vi "Report.vi"() -> ()   [LabVIEW 2017]
uses:
  <vilib>/Utility/miscctls.llb/LVRowAndColumnTypeDef.ctl
  <vilib>/Utility/miscctls.llb/LVRowAndColumnUnsignedTypeDef.ctl
  a160b8e7-0040-4e34-a052-5f80b3aab475.vi
  <vilib>/addons/database/Connection.llb/DB Tools Open Connec (String).vi
  <vilib>/Utility/file.llb/Write Delimited Spreadsheet (string).vi
  Global/Global 1.vi
  <vilib>/regexp/Match Regular Expression.xnode
  <vilib>/addons/database/NI_Database_API.lvlib
  <vilib>/Utility/NIReport.llb/NI_report.lvclass
  <vilib>/Utility/NIReport.llb/Append Text Table to Report (wrap).vi
panel:
  out "reposr save header":string[](array[string])
  in  "SELECT REPORT TYPE":string(combo)="WITH TRECIABILITY"
  out "error out":errorcluster
  in  "error in (no error)":errorcluster
  in  "GET REPORT":bool
  in  "EXIT":bool
  in  "EXPORT TO EXCEL":bool
  in  "TO":timestamp format="%<%x>T"
  in  "FROM":timestamp format="%<%x>T"
  in  "BARCODE":string
  in  "TYPE":string(combo)="DATE TIME"
  in  "STATION WISE":string(combo)="0"
  out "Table":string[][](table)
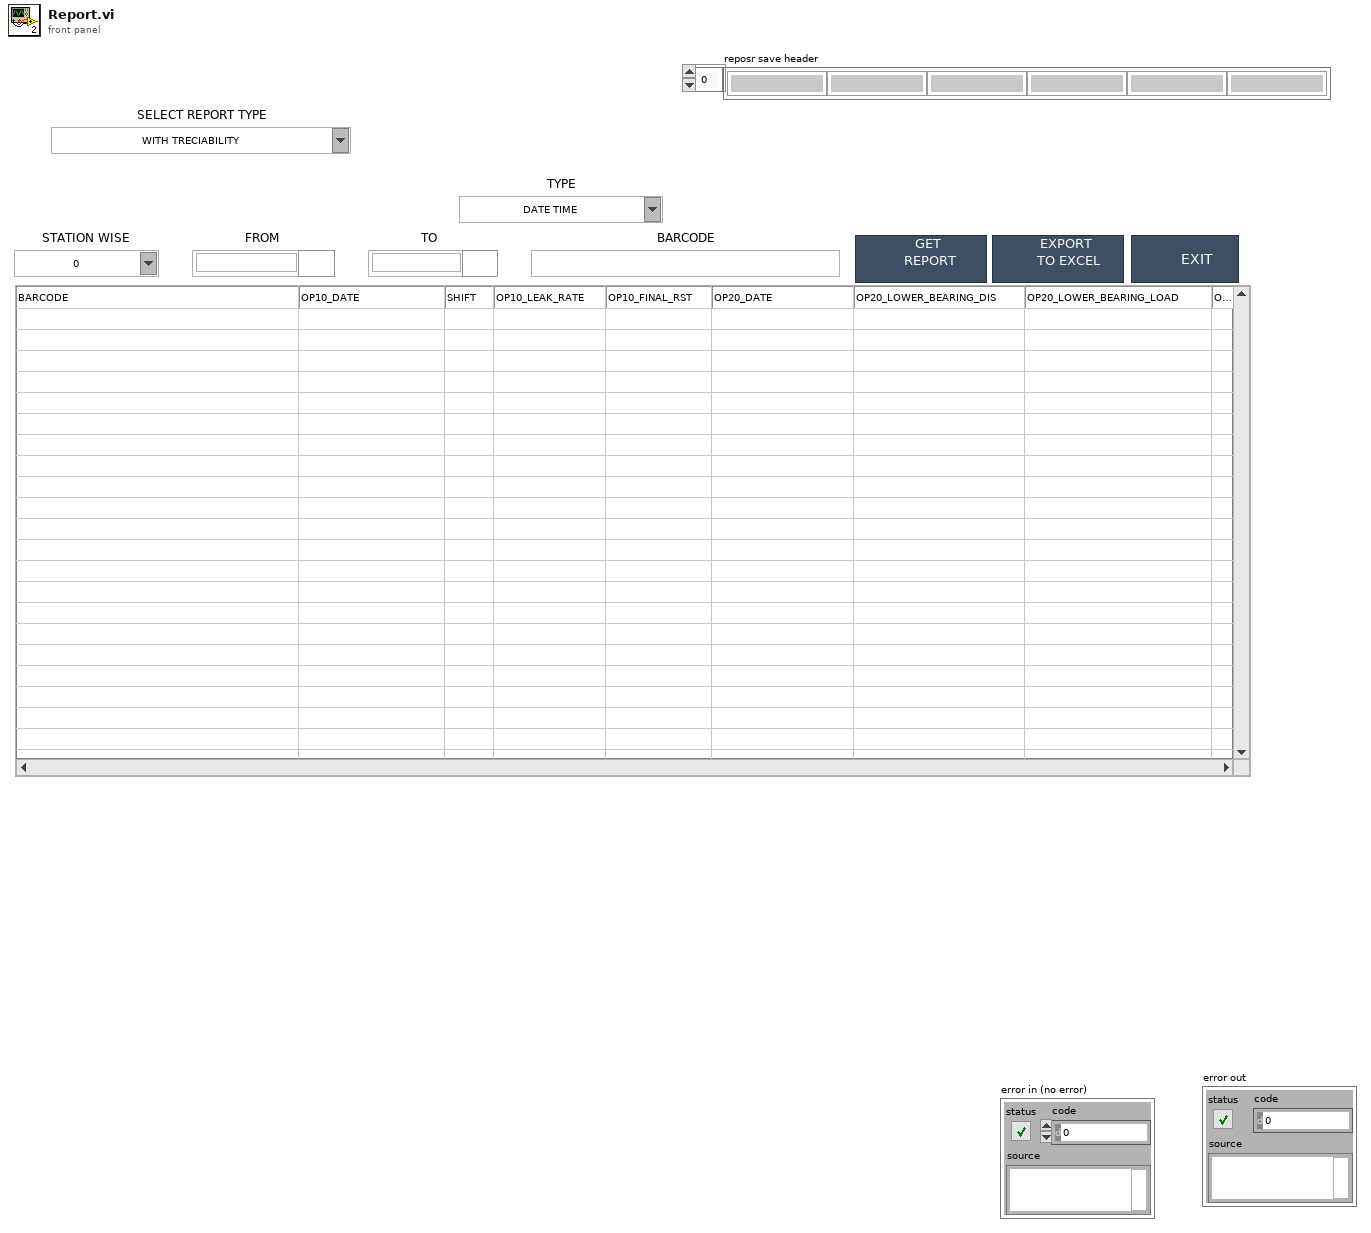
[diagram p1: front panel]
types:
  T1 = typedef "NI_Database_API.lvlib/Conn ObjectReference.ctl" = refnum<k1>
  T2 = typedef "LVRowAndColumnTypeDef.ctl" = cluster{"Row":i32, "Column":i32}
  T3 = typedef "LVRowAndColumnUnsignedTypeDef.ctl" = cluster{"Row":u32, "Column":u32}
  T4 = enum16{"Standard Report", "HTML", "Word", "Excel"}
  T5 = enum16{"maximized", "minimized", "normal", "no change"}
  T6 = enum32{"invalid app kind", "Development System", "Run Time System", "Student Edition", "Embedded LabVIEW", "Evaluation", "Custom"}
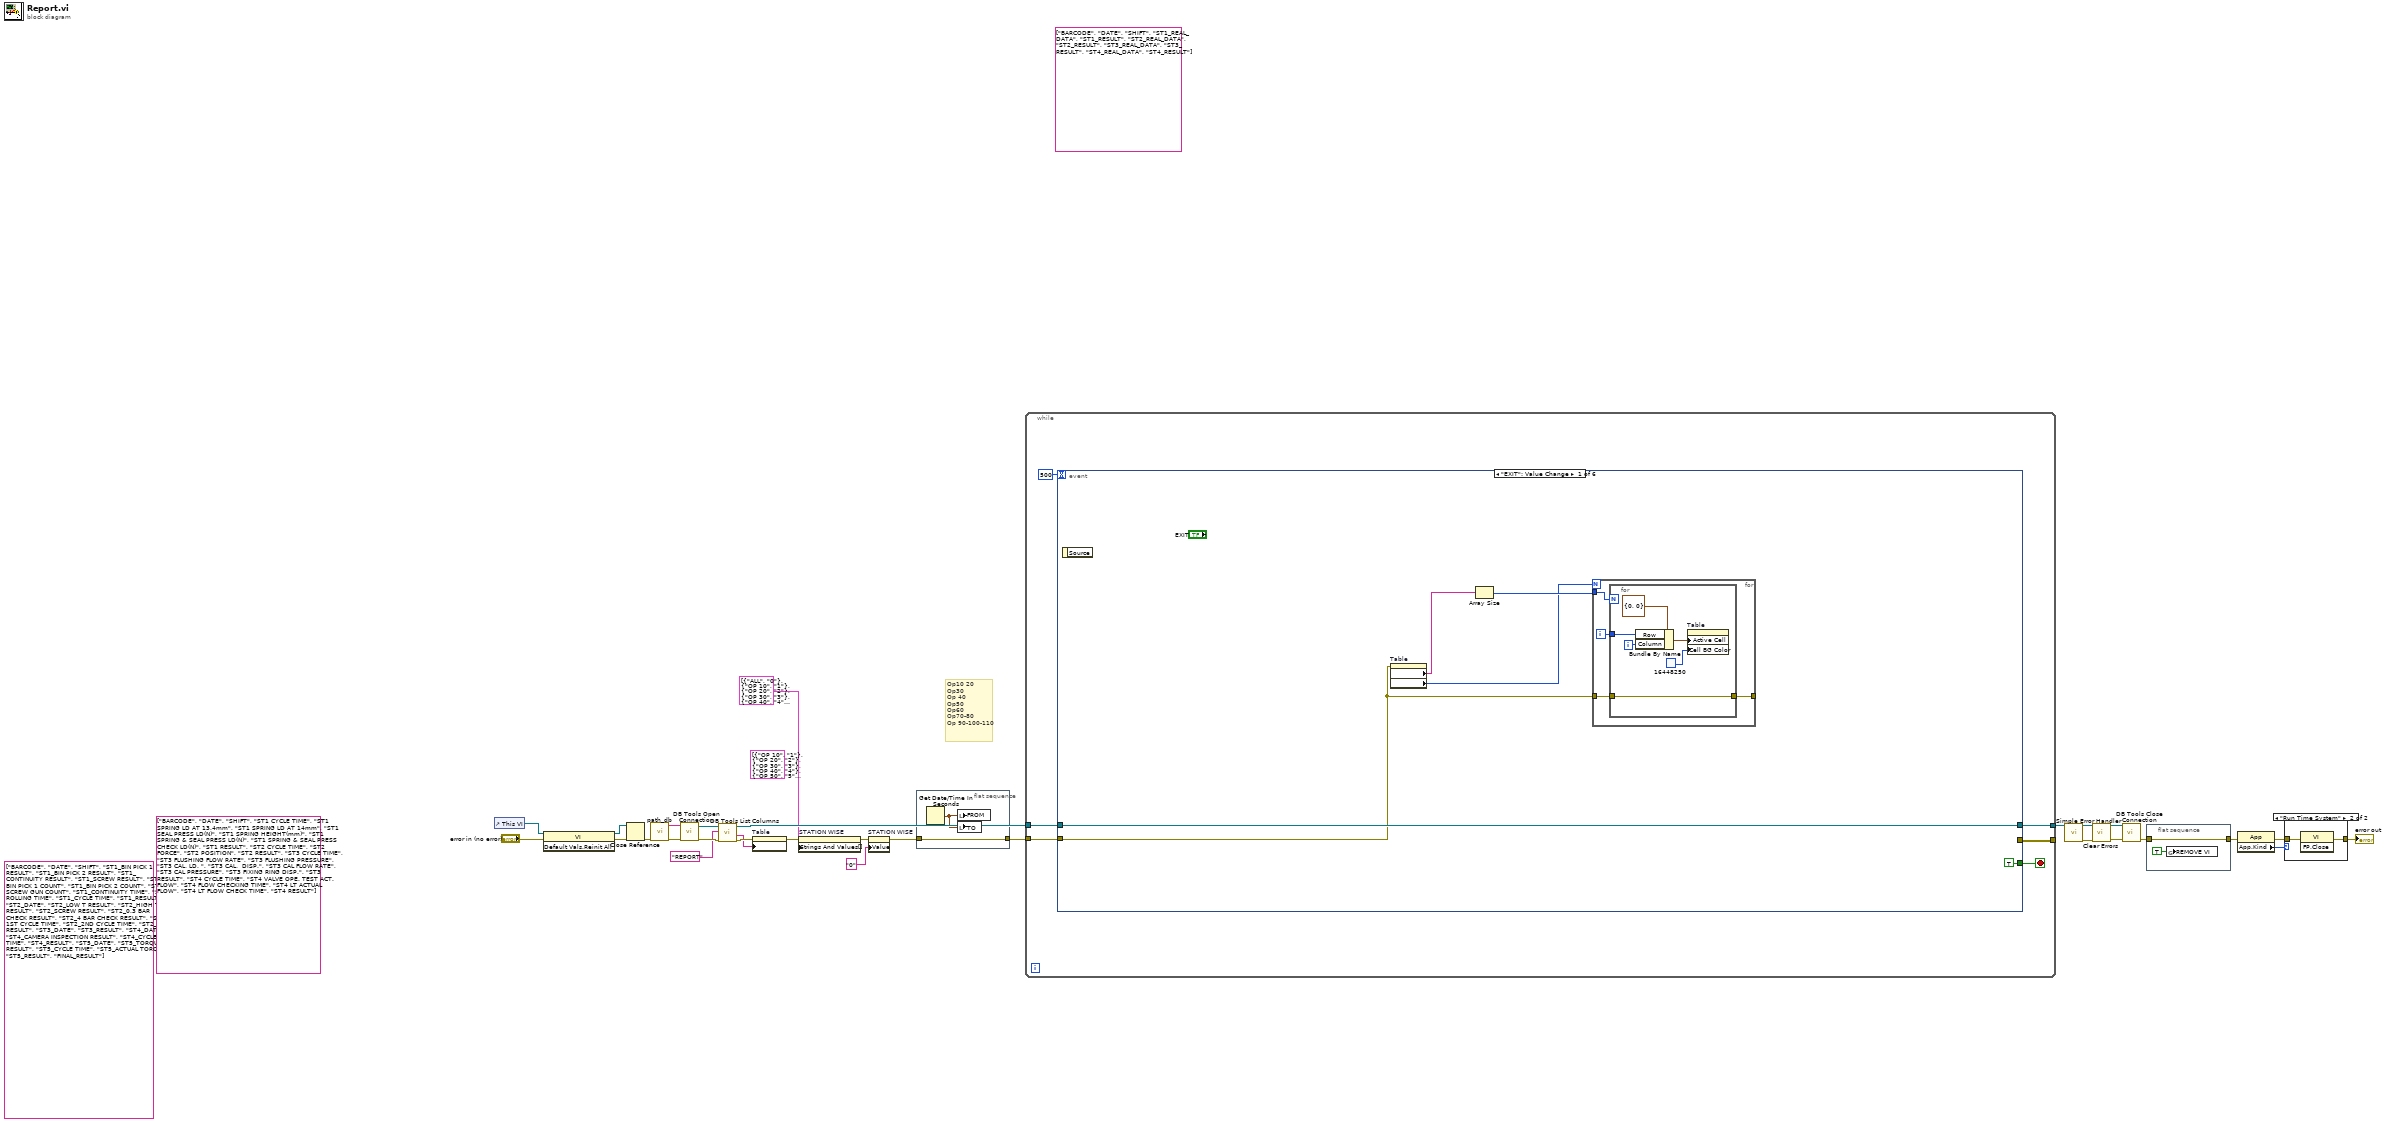
[diagram p0: block diagram]
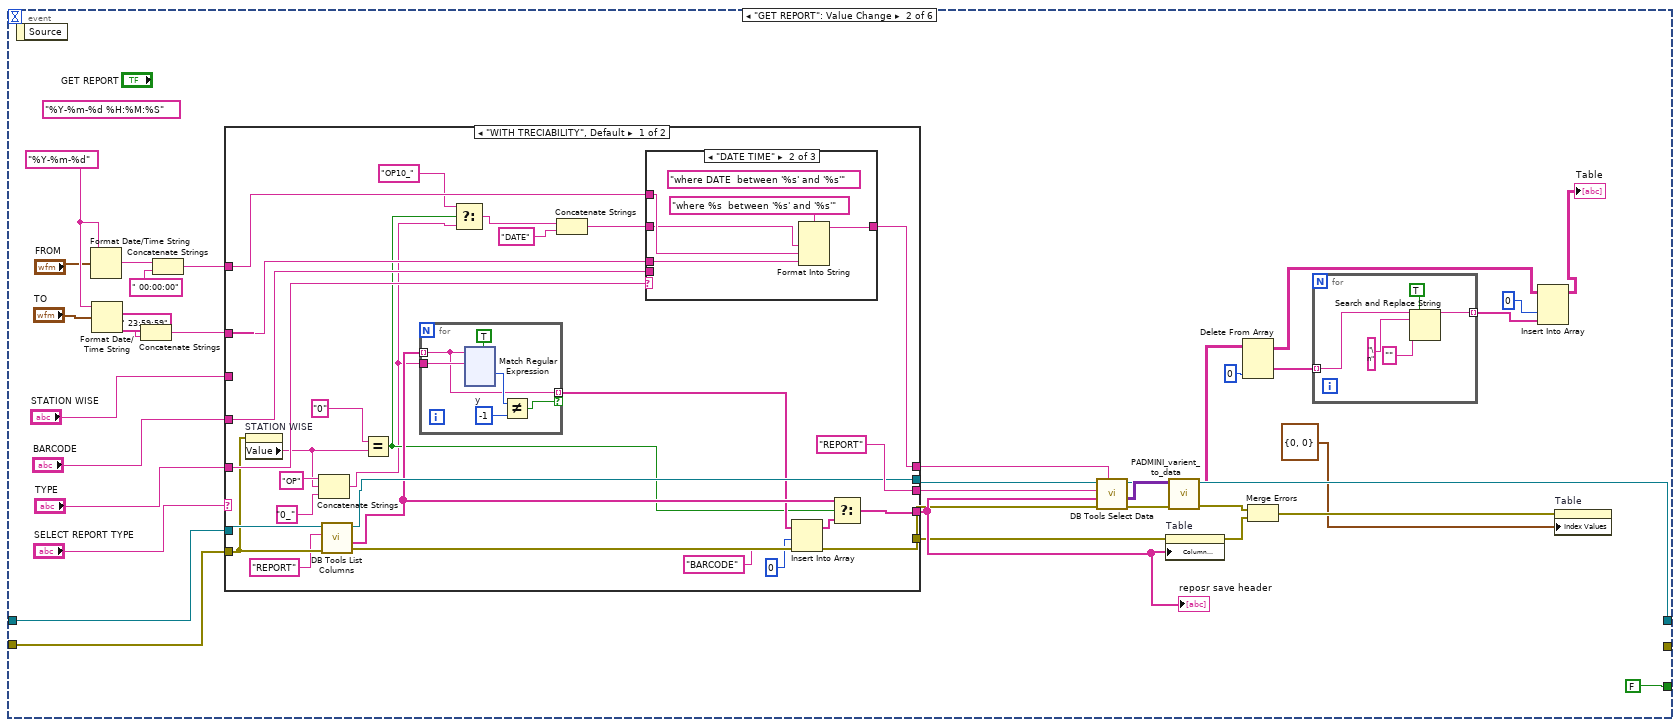
[diagram p2: hidden frame]
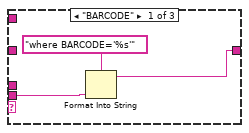
[diagram p3: hidden frame]
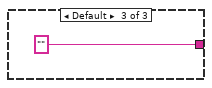
[diagram p4: hidden frame]
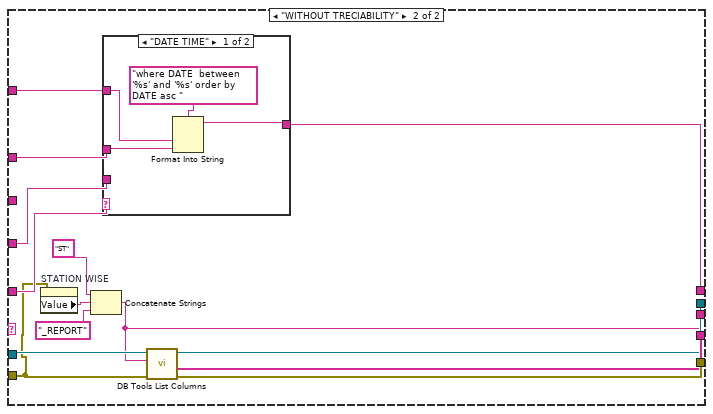
[diagram p5: hidden frame]
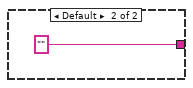
[diagram p6: hidden frame]
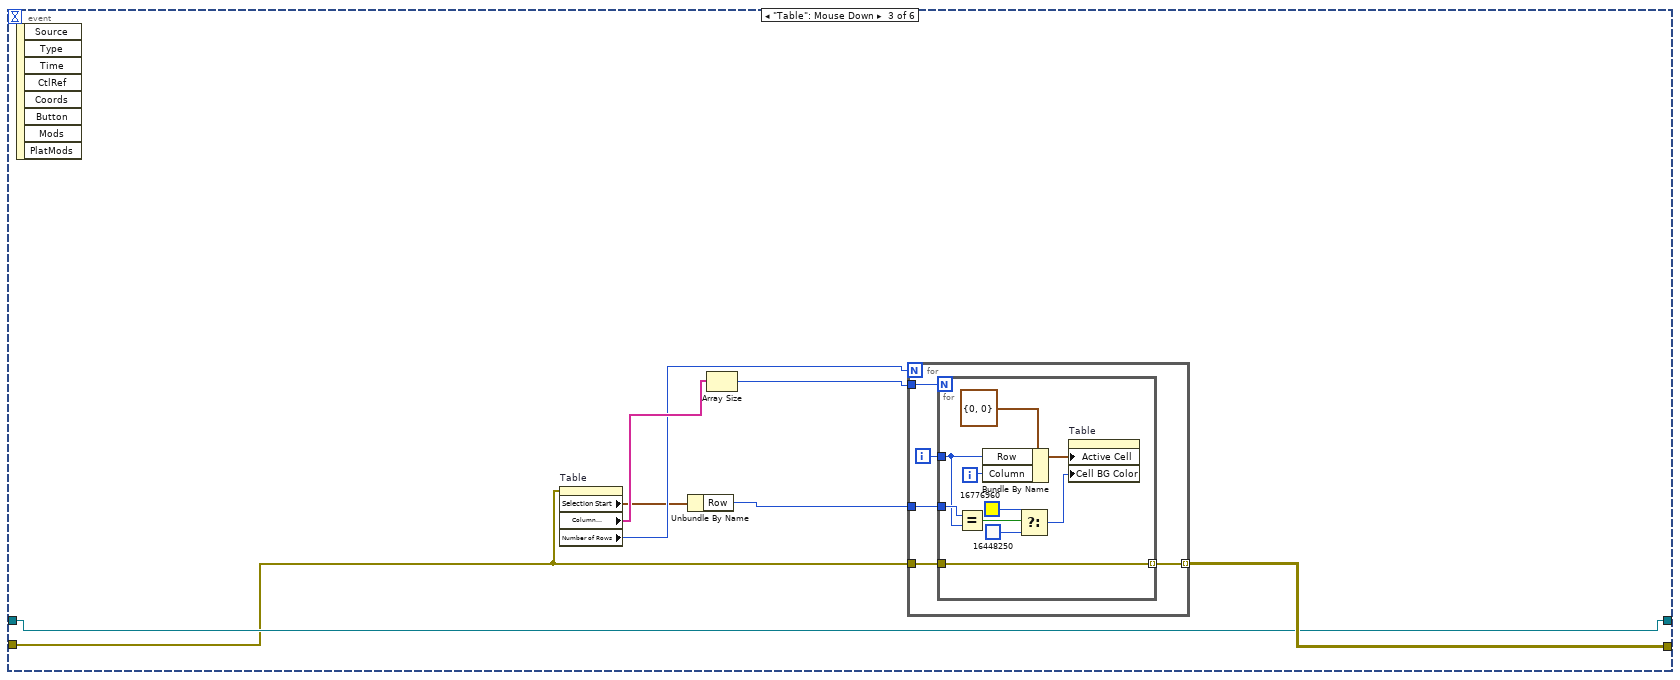
[diagram p7: hidden frame]
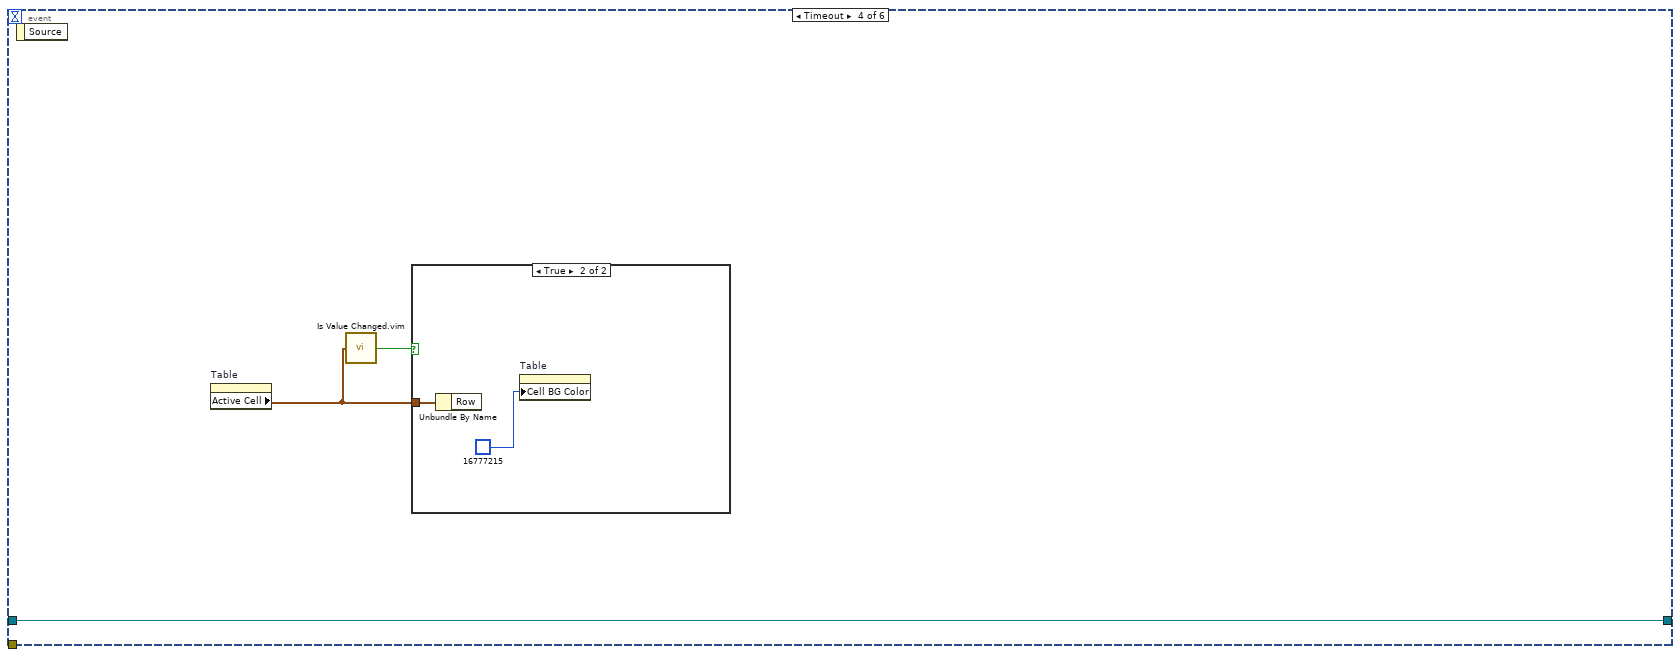
[diagram p8: hidden frame]
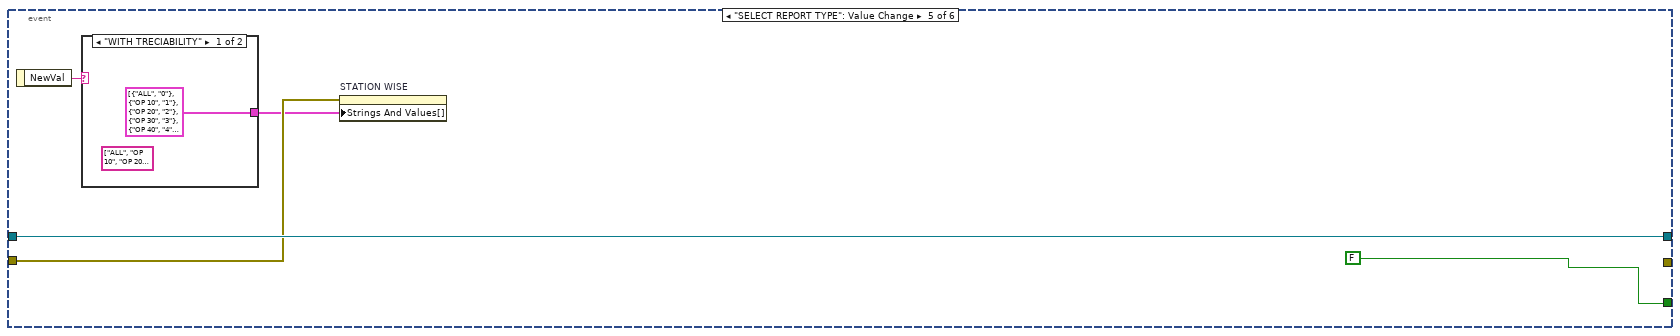
[diagram p10: hidden frame]
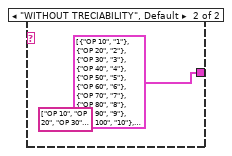
[diagram p11: hidden frame]
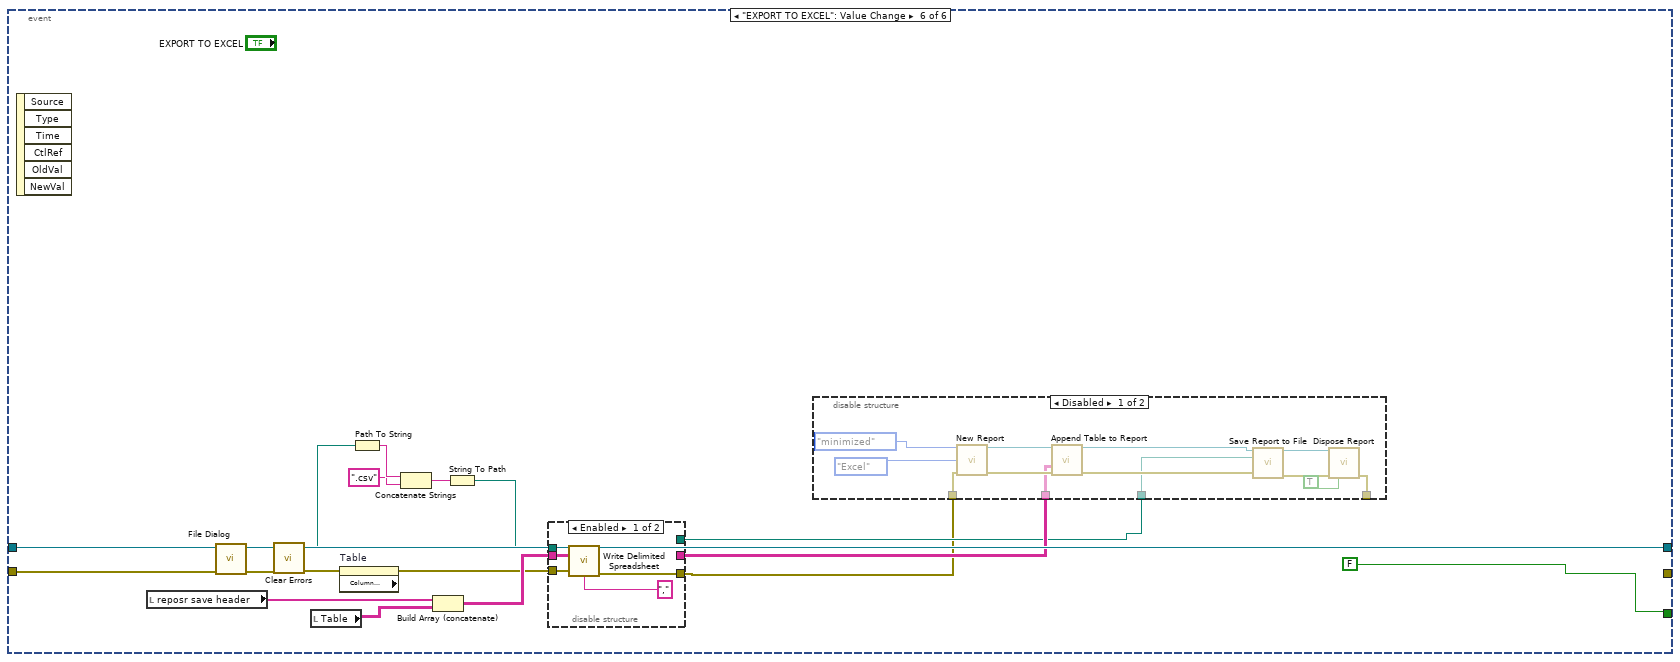
[diagram p12: hidden frame]
diagram:
  (unwired) cluster{"String":string, "Value":string}[] [{"String"="OP 10", "Value"="1"}, {"String"="OP 20", "Value"="2"}, {"String"="OP 30", "Value"="3"}, {"String"="OP 40", "Value"="4"}, {"String"="OP 50", "Value"="5"}, {"String"="OP 60", "Value"="6"}, {"String"="OP 70", "Value"="7"}, {"String"="OP 80", "Value"="8"}, {"String"="OP 90", "Value"="9"}, {"String"="OP 100", "Value"="10"}, {"String"="OP 110", "Value"="11"}] ("Strings And Values [] 2")
  (unwired) string[] ["BARCODE", "DATE", "SHIFT", "ST1_REAL_DATA", "ST1_RESULT", "ST2_REAL_DATA", "ST2_RESULT", "ST3_REAL_DATA", "ST3_RESULT", "ST4_REAL_DATA", "ST4_RESULT"]
  (unwired) string[] ["BARCODE", "DATE", "SHIFT", "ST1_BIN PICK 1 RESULT", "ST1_BIN PICK 2 RESULT", "ST1_CONTINUITY RESULT", "ST1_SCREW RESULT", "ST1_BIN PICK 1 COUNT", "ST1_BIN PICK 2 COUNT", "ST1_SCREW GUN COUNT", "ST1_CONTINUITY TIME", "ST1_ROLLING TIME", "ST1_CYCLE TIME", "ST1_RESULT", "ST2_DATE", "ST2_LOW T RESULT", "ST2_HIGH T RESULT", "ST2_SCREW RESULT", "ST2_0.3 BAR CHECK RESULT", "ST2_4 BAR CHECK RESULT", "ST2_1ST CYCLE TIME", "ST2_2ND CYCLE TIME", "ST2_RESULT", "ST3_DATE", "ST3_RESULT", "ST4_DATE", "ST4_CAMERA INSPECTION RESULT", "ST4_CYCLE TIME", "ST4_RESULT", "ST5_DATE", "ST5_TORQUE RESULT", "ST5_CYCLE TIME", "ST5_ACTUAL TORQUE", "ST5_RESULT", "FINAL_RESULT"]
  (unwired) string[] ["BARCODE", "DATE", "SHIFT", "ST1 CYCLE TIME", "ST1 SPRING LD AT 13.4mm", "ST1 SPRING LD AT 14mm", "ST1 SEAL PRESS LD(N)", "ST1 SPRING HEIGHT(mm)", "ST1 SPRING & SEAL PRESS LD(N)", "ST1 SPRING & SEAL PRESS CHECK LD(N)", "ST1 RESULT", "ST2 CYCLE TIME", "ST2 FORCE", "ST2 POSITION", "ST2 RESULT", "ST3 CYCLE TIME", "ST3 FLUSHING FLOW RATE", "ST3 FLUSHING PRESSURE", "ST3 CAL. LD. ", "ST3 CAL.  DISP.", "ST3 CAL FLOW RATE", "ST3 CAL PRESSURE", "ST3 FIXING RING DISP.", "ST3 RESULT", "ST4 CYCLE TIME", "ST4 VALVE OPE. TEST ACT. FLOW", "ST4 FLOW CHECKING TIME", "ST4 LT ACTUAL FLOW", "ST4 LT FLOW CHECK TIME", "ST4 RESULT"]
  # "Op10 20\nOp30\nOp 40\nOp50\nOp60\nOp70-80\nOp 90-100-110"
  n1 = control-ref of="This VI"() -> (w27:refnum<vi>)
  n2 = invoke class="VI" method="Default Vals.Reinit All"(reference=w27, error in="error in (no error)") -> (reference out=w25:refnum<vi>, error out=w24:errorcluster)  [unwired: 1 in, 1 out]
  n3 = Close Reference(reference=w25, error in (no error)=w24) -> (error out=w15:errorcluster)
  n4 = call "path_db.vi"("error in"=w15) -> ("error out"=w17:errorcluster, "resulting string"=w16:string)  [unwired: 9 in]
  n5 = call-poly <vilib>:"DB Tools Open Connection.vi"("error in (no error)"=w17, "connection information"=w16) -> ("error out"=w10:errorcluster, "connection reference"=w7:T1)  [unwired: 6 in]
  n6 = call <vilib>:"DB Tools List Columns.vi"("error in (no error)"=w10, "table"="REPORT", "connection reference"=w7) -> ("error out"=w9:errorcluster, "columns"=w6:string[], "connection reference out"=w8:T1)  [unwired: 1 in, 1 out]
  n7 = property on="Table" class="Tbl (strict)"(error in=w9, "Column Headers[]"=w6) -> (error out=w12:errorcluster)  [unwired: 1 in, 1 out]
  n8 = property on="STATION WISE" class="CmbBox"(error in=w12, "Strings And Values[]"=cluster{"String":string, "Value":string}[] [{"String"="ALL", "Value"="0"}, {"String"="OP 10", "Value"="1"}, {"String"="OP 20", "Value"="2"}, {"String"="OP 30", "Value"="3"}, {"String"="OP 40", "Value"="4"}, {"String"="OP 50", "Value"="5"}, {"String"="OP 60", "Value"="6"}, {"String"="OP 70", "Value"="7"}, {"String"="OP 80", "Value"="8"}, {"String"="OP 90", "Value"="9"}, {"String"="OP 100", "Value"="10"}, {"String"="OP 110", "Value"="11"}] ("Strings And Values [] 2")) -> (error out=w4:errorcluster)  [unwired: 1 in, 1 out]
  n9 = property on="STATION WISE" class="CmbBox"(error in=w4, "Value"="0") -> (error out=w3:errorcluster)  [unwired: 1 in, 1 out]
  n10 = flat-sequence {
    tunnel: w3 -> [w28]
    tunnel: [w28] -> w11
    frame #0 {
      n11 = Get Date/Time In Seconds() -> (seconds since 1Jan1904=w29:timestamp)
      n12 = local write "FROM"(w29) -> ()
      n13 = local write "TO"(w29) -> ()
    }
  }
  n14 = while {
    tunnel: [w32] -> _
    tunnel: w11 -> [w34]
    tunnel: w8 -> [w33]
    tunnel: [w31] -> w13
    stop <- w35 stop-if-true
    n15 = event shown="[0] \"EXIT\": Value Change" {
      selector: _ -> [_ _ _ _ _ _]
      dyn-events: _ -> [_ _ _ _ _ _]
      timeout: 500 -> [_ _ _ _ _ _]
      tunnel: [TRUE FALSE _ _ FALSE FALSE] -> w35
      tunnel: w34 -> [w36 w64 w267 _ w297 w306]
      tunnel: w33 -> [w40 w62 w273 w292 w299 w317]
      tunnel: [w40 w70 w273 w292 w299 w317] -> w31
      tunnel: [_ _ w274 _ _ _] -> w32
      event "EXIT": Value Change {
        n16 = event-data() -> ()  [unwired: 1 in, 1 out]
        n17 = property on="Table" class="Tbl (strict)"(error in=w36) -> ("Column Headers[]"=w39:string[], "Number of Rows"=w37:u32)  [unwired: 1 in, 2 out]
        n18 = Array Size(array=w39) -> (size(s)=w38:i32)
        n19 = for {
          N: w37 -> [_]
          tunnel: w38 -> [w45]
          tunnel: [w42] -> _
          tunnel: w36 -> [w43]
          i -> [w44]
          n20 = for {
            N: w45 -> [_]
            tunnel: w44 -> [w48]
            tunnel: w43 -> [w47]
            tunnel: [w47] -> w42
            i -> [w49]
            n21 = Bundle By Name(cluster=T2 {"Row"=0, "Column"=0} ("Selection Start 2"), "Row"=w48, "Column"=w49) -> (w50:T2)
            n22 = property on="Table" class="Tbl (strict)"("Active Cell"=w50, "Cell BG Color"=u32 16448250) -> ()  [unwired: 2 in, 2 out]
          }
        }
      }
      event "GET REPORT": Value Change {
        (unwired) "%Y-%m-%d %H:%M:%S" ("time format string (%c)")
        w83 = "%Y-%m-%d" ("time format string (%c)")
        n23 = event-data() -> ()  [unwired: 1 in, 1 out]
        n24 = Format Date/Time String(time format string (%c)=w83, seconds (now)="FROM") -> (date/time string=w77:string)  [unwired: 1 in]
        n25 = Format Date/Time String(time format string (%c)=w83, seconds (now)="TO") -> (date/time string=w74:string)  [unwired: 1 in]
        n26 = Concatenate Strings(w74, " 23:59:59" ("time format string (%c)")) -> (w73:string)
        n27 = Concatenate Strings(w77, " 00:00:00" ("time format string (%c)")) -> (w76:string)
        n28 = case shown="\"WITH TRECIABILITY\", Default" "SELECT REPORT TYPE" {
          tunnel: "TYPE" -> [w118 w261]
          tunnel: [w117 w260] -> w85
          tunnel: "BARCODE" -> [w116 w259]
          tunnel: w76 -> [w115 w258]
          tunnel: w73 -> [w100 w254]
          tunnel: "STATION WISE" -> [_ _]
          tunnel: ["REPORT" w249] -> w65
          tunnel: w64 -> [w106 w248]
          tunnel: [w111 w253] -> w59
          tunnel: [w98 w252] -> w63
          tunnel: w62 -> [w113 w251]
          tunnel: [w112 w250] -> w61
          frame "WITH TRECIABILITY", Default {
            n29 = property on="STATION WISE" class="CmbBox"(error in=w106) -> ("Value"=w101:string)  [unwired: 1 in, 2 out]
            n30 = Concatenate Strings("OP" ("element"), w101, "0_" ("element")) -> (w93:string)
            n31 = call <vilib>:"DB Tools List Columns.vi"("error in (no error)"=w106, "table"="REPORT", "connection reference"=w113) -> ("error out"=w111:errorcluster, "columns"=w105:string[], "connection reference out"=w112:T1)  [unwired: 1 in, 1 out]
            n32 = Equal?(x="0", y=w101) -> (x = y?=w95:bool)
            n33 = for {
              tunnel: w105 -> [w120] mode=indexing
              tunnel: w93 -> [w124]
              tunnel: [w120] -> w99 mode=indexing if=w119
              w121 = -1  # y
              n34 = xnode "Match Regular Expression"("input string"=w120, "regular expression"=w124, "multiline? (F)"=TRUE) -> ("offset past match"=w122:i32)  [unwired: 3 in, 4 out]
              n35 = Not Equal?(x=w122, y=w121) -> (x != y?=w119:bool)
            }
            n36 = Select(t="OP10_", s=w95, f=w93) -> (s? t:f=w92:string)
            n37 = Concatenate Strings(w92, "DATE") -> (w96:string)
            n38 = case shown="\"DATE TIME\"" w118 {
              tunnel: [w240 w245 ""] -> w117
              tunnel: w116 -> [w239 _ _]
              tunnel: w115 -> [_ w244 _]
              tunnel: w100 -> [_ w243 _]
              tunnel: w96 -> [_ w242 _]
              frame "BARCODE" {
                n39 = Format Into String(format string="where BARCODE='%s'", w239) -> (resulting string=w240:string)  [unwired: 2 in, 1 out]
              }
              frame "DATE TIME" {
                (unwired) "where DATE  between '%s' and '%s'"
                n40 = Format Into String(format string="where %s  between '%s' and '%s'", w242, w244, w243) -> (resulting string=w245:string)  [unwired: 2 in, 1 out]
              }
              frame Default {
              }
            }
            n41 = Insert Into Array(array=w99, index=0, new element="BARCODE" ("String")) -> (w109:string[])
            n42 = Select(t=w105, s=w95, f=w109) -> (s? t:f=w98:string[])
          }
          frame "WITHOUT TRECIABILITY" {
            n43 = property on="STATION WISE" class="CmbBox"(error in=w248) -> ("Value"=w257:string)  [unwired: 1 in, 2 out]
            n44 = Concatenate Strings("ST", w257, "_REPORT") -> (w249:string)
            n45 = case shown="\"DATE TIME\"" w261 {
              tunnel: [w265 ""] -> w260
              tunnel: w259 -> [_ _]
              tunnel: w258 -> [w264 _]
              tunnel: w254 -> [w263 _]
              frame "DATE TIME" {
                n46 = Format Into String(format string="where DATE  between '%s' and '%s' order by DATE asc ", w264, w263) -> (resulting string=w265:string)  [unwired: 2 in, 1 out]
              }
              frame Default {
              }
            }
            n47 = call <vilib>:"DB Tools List Columns.vi"("error in (no error)"=w248, "table"=w249, "connection reference"=w251) -> ("error out"=w253:errorcluster, "columns"=w252:string[], "connection reference out"=w250:T1)  [unwired: 1 in, 1 out]
          }
        }
        "reposr save header" <- w63
        n48 = call <vilib>:"DB Tools Select Data.vi"("condition"=w85, "error in (no error)"=w59, "columns"=w63, "table"=w65, "connection reference"=w61) -> ("error out"=w68:errorcluster, "data"=w72:variant[][], "connection reference out"=w70:T1)  [unwired: 1 in]
        n49 = property on="Table" class="Tbl (strict)"(error in=w59, "Column Headers[]"=w63) -> (error out=w67:errorcluster)  [unwired: 1 in, 1 out]
        n50 = call "PADMINI_varient_to_data.vi"("error in (no error)"=w68, "data"=w72) -> ("error out"=w66:errorcluster, "Array"=w54:string[][])  [unwired: 8 in]
        n51 = Delete From Array(array=w54, index (col)=0 ("disabled index (col)")) -> (deleted portion=w57:string[], array with subset deleted=w55:string[][])  [unwired: 2 in]
        n52 = Merge Errors(w66, w67) -> (w71:errorcluster)
        n53 = for {
          tunnel: w57 -> [w88] mode=indexing
          tunnel: [w87] -> w56 mode=indexing
          n54 = Search and Replace String(replace all?=TRUE ("replace all? (F)"), input string=w88, search string="\n", replace string="" ("replace string (\"\")")) -> (result string=w87:string)  [unwired: 4 in, 3 out]
        }
        n55 = Insert Into Array(array=w55, index (col)=0 ("disabled index (col)"), new element=w56) -> (→"Table":string[][])  [unwired: 1 in]
        n56 = property on="Table" class="Tbl (strict)"(error in=w71, "Index Values"=T3 {"Row"=0, "Column"=0}) -> ()  [unwired: 1 in, 2 out]
      }
      event "Table": Mouse Down {
        n57 = event-data() -> ()  [unwired: 1 in, 8 out]
        n58 = property on="Table" class="Tbl (strict)"(error in=w267) -> ("Selection Start"=w268:T2, "Column Headers[]"=w272:string[], "Number of Rows"=w270:u32)  [unwired: 1 in, 2 out]
        n59 = Unbundle By Name(w268) -> ("Row"=w269:i32)
        n60 = Array Size(array=w272) -> (size(s)=w271:i32)
        n61 = for {
          N: w270 -> [_]
          tunnel: w269 -> [w277]
          tunnel: w271 -> [w279]
          tunnel: [w275] -> w274 mode=indexing
          tunnel: w267 -> [w276]
          i -> [w278]
          n62 = for {
            N: w279 -> [_]
            tunnel: w278 -> [w285]
            tunnel: w277 -> [w286]
            tunnel: w276 -> [w280]
            tunnel: [w280] -> w275 mode=indexing
            i -> [w287]
            n63 = Equal?(x=w286, y=w285) -> (x = y?=w284:bool)
            n64 = Bundle By Name(cluster=T2 {"Row"=0, "Column"=0} ("Selection Start 2"), "Row"=w285, "Column"=w287) -> (w288:T2)
            n65 = Select(t=u32 16776960, s=w284, f=u32 16448250) -> (s? t:f=w281:u32)
            n66 = property on="Table" class="Tbl (strict)"("Active Cell"=w288, "Cell BG Color"=w281) -> ()  [unwired: 2 in, 2 out]
          }
        }
      }
      event Timeout {
        n67 = event-data() -> ()  [unwired: 1 in, 1 out]
        n68 = property on="Table" class="Tbl (strict)"() -> ("Active Cell"=w291:T2)  [unwired: 2 in, 2 out]
        n69 = call "Is Value Changed.vim"("value"=w291) -> ("changed or first call?"=w290:bool)
        n70 = case shown="True" w290 {
          tunnel: w291 -> [_ w294]
          frame False {
          }
          frame True {
            n71 = Unbundle By Name(w294) -> ()  [unwired: 1 out]
            n72 = property on="Table" class="Tbl (strict)"("Cell BG Color"=u32 16777215) -> ()  [unwired: 2 in, 2 out]
          }
        }
      }
      event "SELECT REPORT TYPE": Value Change {
        n73 = event-data() -> ("NewVal"=w298:string)  [unwired: 1 in]
        n74 = case shown="\"WITH TRECIABILITY\"" w298 {
          tunnel: [cluster{"String":string, "Value":string}[] [{"String"="ALL", "Value"="0"}, {"String"="OP 10", "Value"="1"}, {"String"="OP 20", "Value"="2"}, {"String"="OP 30", "Value"="3"}, {"String"="OP 40", "Value"="4"}, {"String"="OP 50", "Value"="5"}, {"String"="OP 60", "Value"="6"}, {"String"="OP 70", "Value"="7"}, {"String"="OP 80", "Value"="8"}, {"String"="OP 90", "Value"="9"}, {"String"="OP 100", "Value"="10"}, {"String"="OP 110", "Value"="11"}] ("Strings And Values [] 2") cluster{"String":string, "Value":string}[] [{"String"="OP 10", "Value"="1"}, {"String"="OP 20", "Value"="2"}, {"String"="OP 30", "Value"="3"}, {"String"="OP 40", "Value"="4"}, {"String"="OP 50", "Value"="5"}, {"String"="OP 60", "Value"="6"}, {"String"="OP 70", "Value"="7"}, {"String"="OP 80", "Value"="8"}, {"String"="OP 90", "Value"="9"}, {"String"="OP 100", "Value"="10"}, {"String"="OP 110", "Value"="11"}] ("Strings And Values [] 2")] -> w295
          frame "WITH TRECIABILITY" {
            (unwired) string[] ["ALL", "OP 10", "OP 20", "OP 30", "OP 40", "OP 50", "OP 60", "OP 70", "OP 80", "OP 90", "OP 100", "OP 110"] ("Strings []")
          }
          frame "WITHOUT TRECIABILITY", Default {
            (unwired) string[] ["OP 10", "OP 20", "OP 30", "OP 40", "OP 50", "OP 60", "OP 70", "OP 80", "OP 90", "OP 100", "OP 110"] ("Strings []")
          }
        }
        n75 = property on="STATION WISE" class="CmbBox"(error in=w297, "Strings And Values[]"=w295) -> ()  [unwired: 1 in, 2 out]
      }
      event "EXPORT TO EXCEL": Value Change {
        n76 = event-data() -> ()  [unwired: 1 in, 6 out]
        n77 = local read "reposr save header"() -> (w302:string[])
        n78 = call "File Dialog"("error in"=w306) -> ("selected path"=w315:path, "error out"=w316:errorcluster)  [unwired: 11 in, 2 out]
        n79 = call <vilib>:"Clear Errors.vi"("error in (no error)"=w316) -> ("error out"=w309:errorcluster)  [unwired: 5 in, 1 out]
        n80 = local read "Table"() -> (w318:string[][])
        n81 = property on="Table" class="Tbl (strict)" props=["Column Headers[]"](error in=w309) -> (error out=w308:errorcluster)  [unwired: 1 in, 2 out]
        n82 = Path To String(path=w315) -> (string=w314:string)
        n83 = Concatenate Strings(w314, ".csv" ("string")) -> (w312:string)
        n84 = Build Array (concatenate)(w302, w318) -> (w310:string[][])
        n85 = String To Path(string=w312) -> (path=w311:path)
        n86 = disable-structure shown="Enabled" {
          disable-tunnel: w311 -> [w337 w338]
          disable-tunnel: [w336 w340] -> w303
          disable-tunnel: w310 -> [w335 w339]
          disable-tunnel: w308 -> [w333 w340]
          disable-tunnel: [_ w339] -> w305
          disable-tunnel: [_ w338] -> w304
          frame Enabled {
            n87 = call-poly <vilib>:"Write Delimited Spreadsheet.vi"("file path (dialog if empty)"=w337, "2D data"=w335, "error in (no error)"=w333, "delimiter (\\t)"="," ("delimiter (\\t)")) -> ("error out"=w336:errorcluster)  [unwired: 10 in, 1 out]
          }
          frame Disabled {
          }
        }
        n88 = disable-structure shown="Disabled" {
          disable-tunnel: w305 -> [w322 _]
          disable-tunnel: w304 -> [w321 _]
          disable-tunnel: [w320 w332] -> _
          disable-tunnel: w303 -> [w319 w332]
          frame Disabled {
            n89 = call <vilib>:"New Report.vi"("window state (normal)"=T5."minimized", "report type"=T4."Excel", "error in (no error)"=w319) -> ("report out"=w329:refnum<class "NI_report.lvclass">, "error out"=w328:errorcluster)  [unwired: 11 in]
            n90 = call-poly <vilib>:"Append Table to Report.vi"("report in"=w329, "text data"=w322, "error in (no error)"=w328) -> ("report out"=w325:refnum<class "NI_report.lvclass">, "error out"=w327:errorcluster)  [unwired: 9 in, 2 out]
            n91 = call-dynamic "Save Report to File.vi"("report in"=w325, "report file path"=w321, "error in (no error)"=w327) -> ("report out"=w324:refnum<class "NI_report.lvclass">, "error out"=w326:errorcluster)  [unwired: 11 in]
            n92 = call-dynamic "Dispose Report.vi"("report in"=w324, "error in (no error)"=w326, "close report? (T)"=TRUE) -> ("error out"=w320:errorcluster)  [unwired: 12 in]
          }
          frame Enabled {
          }
        }
      }
    }
  }
  n93 = call <vilib>:"Simple Error Handler.vi"() -> ("error out"=w23:errorcluster)  [unwired: 5 in, 4 out]
  n94 = call <vilib>:"Clear Errors.vi"("error in (no error)"=w23) -> ("error out"=w22:errorcluster)  [unwired: 5 in, 1 out]
  n95 = call <vilib>:"DB Tools Close Connection.vi"("error in (no error)"=w22, "connection reference"=w13) -> ("error out"=w14:errorcluster)  [unwired: 5 in]
  n96 = flat-sequence {
    tunnel: [w342] -> w21
    tunnel: w14 -> [w342]
    frame #0 {
      n97 = global write "Global 1.vi" "REMOVE VI"(TRUE ("REMOVE VI")) -> ()
    }
  }
  n98 = property class="App"(error in=w21) -> (error out=w20:errorcluster, "App.Kind"=w19:T6)  [unwired: 1 in, 1 out]
  n99 = case shown="\"Run Time System\"" w19 {
    tunnel: w20 -> [w343 w345]
    tunnel: [w343 w344] -> w18
    frame "Development System", Default {
    }
    frame "Run Time System" {
      n100 = invoke class="VI" method="FP.Close"(error in=w345) -> (error out=w344:errorcluster)  [unwired: 2 in, 2 out]
    }
  }
  "error out" <- w18
